vi "rmx13_tx - Copy (2).vi"() -> ()   [LabVIEW 2012]
uses:
  <vilib>/robotics/Steering/Steering Frame/NI_Robotics_Steering Frame.lvclass
  <vilib>/robotics/Steering/Wheel/NI_Robotics_Wheel.lvclass
  <vilib>/robotics/Utilities/Visualization/Steering Visualization/Steering Picture/NI_Robotics_Steering Picture.lvlib
  <vilib>/robotics/Steering/Fixed Wheel/Create Fixed Wheel.vi
  <vilib>/robotics/Steering/Fixed Wheel/NI_Robotics_Fixed Wheel.lvclass
  <vilib>/robotics/Steering/Differential Steering Frame/Create Differential Steering Frame.vi
  <vilib>/robotics/Steering/Differential Steering Frame/NI_Robotics_Differential Steering Frame.lvclass
  <vilib>/Utility/inputDevices.llb/closeKeyboard.vi
  <vilib>/robotics/Steering/Steering Frame/Apply Steering Frame Velocity to Wheels.vi
  <vilib>/Utility/inputDevices.llb/keyboardAcquire.vi
  <vilib>/robotics/Steering/Wheel/Wheel Parameters.ctl
  <vilib>/robotics/Steering/Wheel/Rotation Direction.ctl
panel:
  in  "Tab Control":enum32{"Front Panel", "Error Control"}(tab)
  in  "Boolean 2":bool
  in  "Boolean":bool
  out "Total Elapsed Time  (HH:MM:SS)":dbl format="%<%H:%M:%S%2u>t"
  out "hup":bool
  out "hdown":bool
  out "xfwd":bool
  out "xback":bool
  out "xdown":bool
  out "xup":bool
  out "right":bool
  out "left":bool
  out "down":bool
  out "up":bool
  out "right motor":dbl(knob) scale=-255.0..255.0
  out "left motor":dbl(knob) scale=-255.0..255.0
  out "Right":dbl=7.0 format="%#.2g"
  out "Left":dbl=3.0 format="%#.2g"
  out "picture":picture
  out "x-dir":string="a"
  out "bot-dir":string="a"
  out "x-state":string="a"
  out "h-state":string="a"
  out "error out":errorcluster
  in  "Horizontal Axis AI Pin":u8
  out "Out":dbl
  out "tx_string":string
  out "bytes written":i32
  # "Left Motor"
  # "Right Motor"
  # "Excavator State"
  # "Excavator Direction"
  # "Elapsed Time"
  # "Start/Stop"
  # "Bot Direction"
  # "Hopper State"
  # "Dump Position"
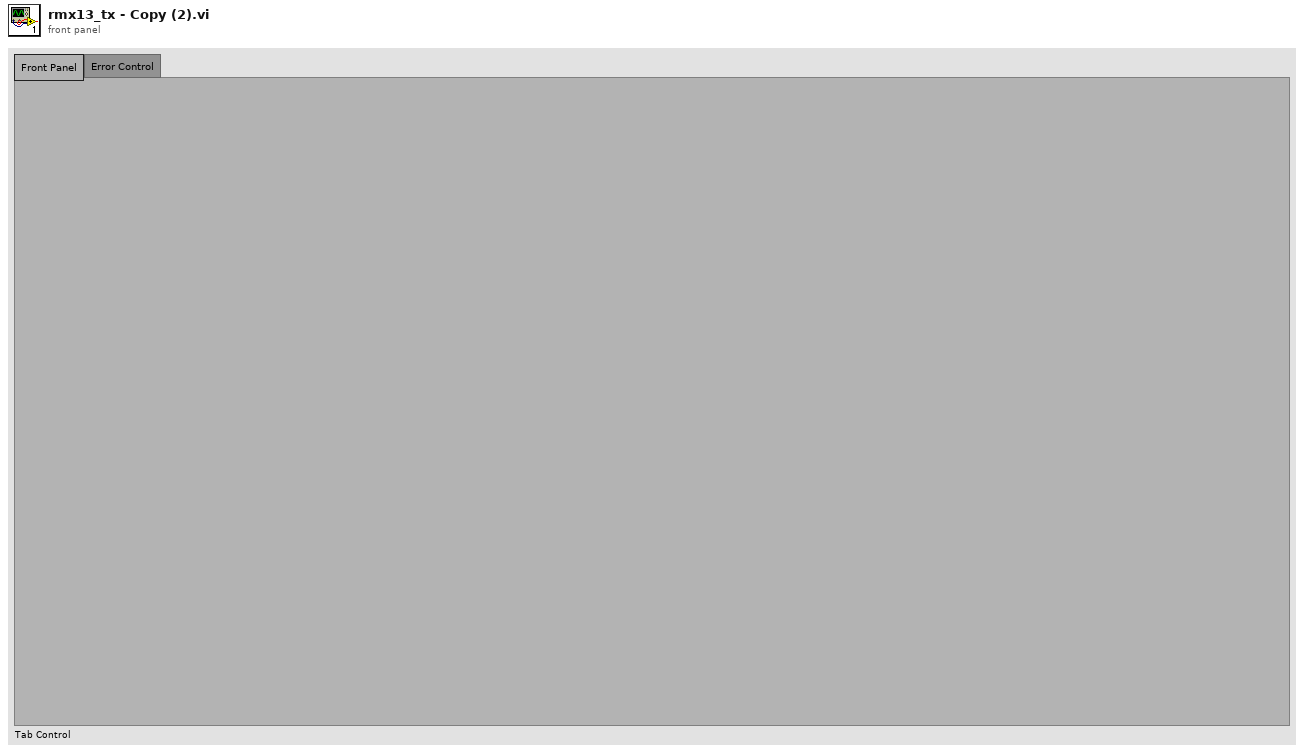
[diagram p1: front panel]
types:
  T1 = typedef "NI_Robotics_Wheel.lvclass/Wheel Parameters.ctl" = cluster{"wheel radius":dbl, "gear ratio":dbl, "forward rotation direction":T2}
  T2 = typedef "NI_Robotics_Wheel.lvclass/Rotation Direction.ctl" = u16
  T3 = cluster{"fixed wheel out":refnum<class "NI_Robotics_Fixed Wheel.lvclass">, "fixed wheel out":refnum<class "NI_Robotics_Fixed Wheel.lvclass">}
  T4 = typedef "LVBoundsTypeDef.ctl" = cluster{"Width":u32, "Height":u32}
  T5 = enum16{"0", "1", "2", "3", "4", "5", "6", "7", "8", "9", "A", "B", "C", "D", "E", "F", "G", "H", "I", "J", "K", "L", "M", "N", "O", "P", "Q", "R", "S", "T", "U", "V", "W", "X", "Y", "Z", "F1", "F2", "F3", "F4", "F5", "F6", "F7", "F8", "F9", "F10", "F11", "F12", "F13", "F14", "F15", "ADD", "BACK", "BACKSLASH", "CAPITAL", "COMMA", "DECIMAL", "DELETE", "DIVIDE", "DOWN", "END", "EQUALS", "ESCAPE", "GRAVE (`)", "HOME", "INSERT", "LBRACKET", "LCONTROL", "LEFT", "L ALT", "LSHIFT", "LWIN", "MINUS", "MULTIPLY", "NEXT", "NUMLOCK", "NUMPAD_0", "NUMPAD_1", "NUMPAD_2", "NUMPAD_3", "NUMPAD_4", "NUMPAD_5", "NUMPAD_6", "NUMPAD_7", "NUMPAD_8", "NUMPAD_9", "PAUSE", "PERIOD", "PRIOR (PG UP)", "RBRACKET", "RCONTROL", "RETURN", "RIGHT", "R ALT", "RSHIFT", "RWIN", "SCROLL", "SEMICOLON", "SLASH", "SPACE", "SUBTRACT", "TAB", "UP", "ENTER (num pad)", "' (quote)"}[]
  T6 = cluster{"up":bool, "down":bool, "left":bool, "right":bool, "xup":bool, "xdown":bool, "hup":bool, "hdown":bool, "xfwd":bool, "xback":bool}
  T7 = cluster{"bot_dir":string, "x-state":string, "h-state":string, "x-dir":string}
  T8 = typedef "NI_Robotics_Wheel.lvclass/Wheel State.ctl" = cluster{"wheel name":string, "forward angular velocity":dbl, "caster angular velocity":dbl, "caster wheel angle (rad)":dbl, "steering angle (rad)":dbl}
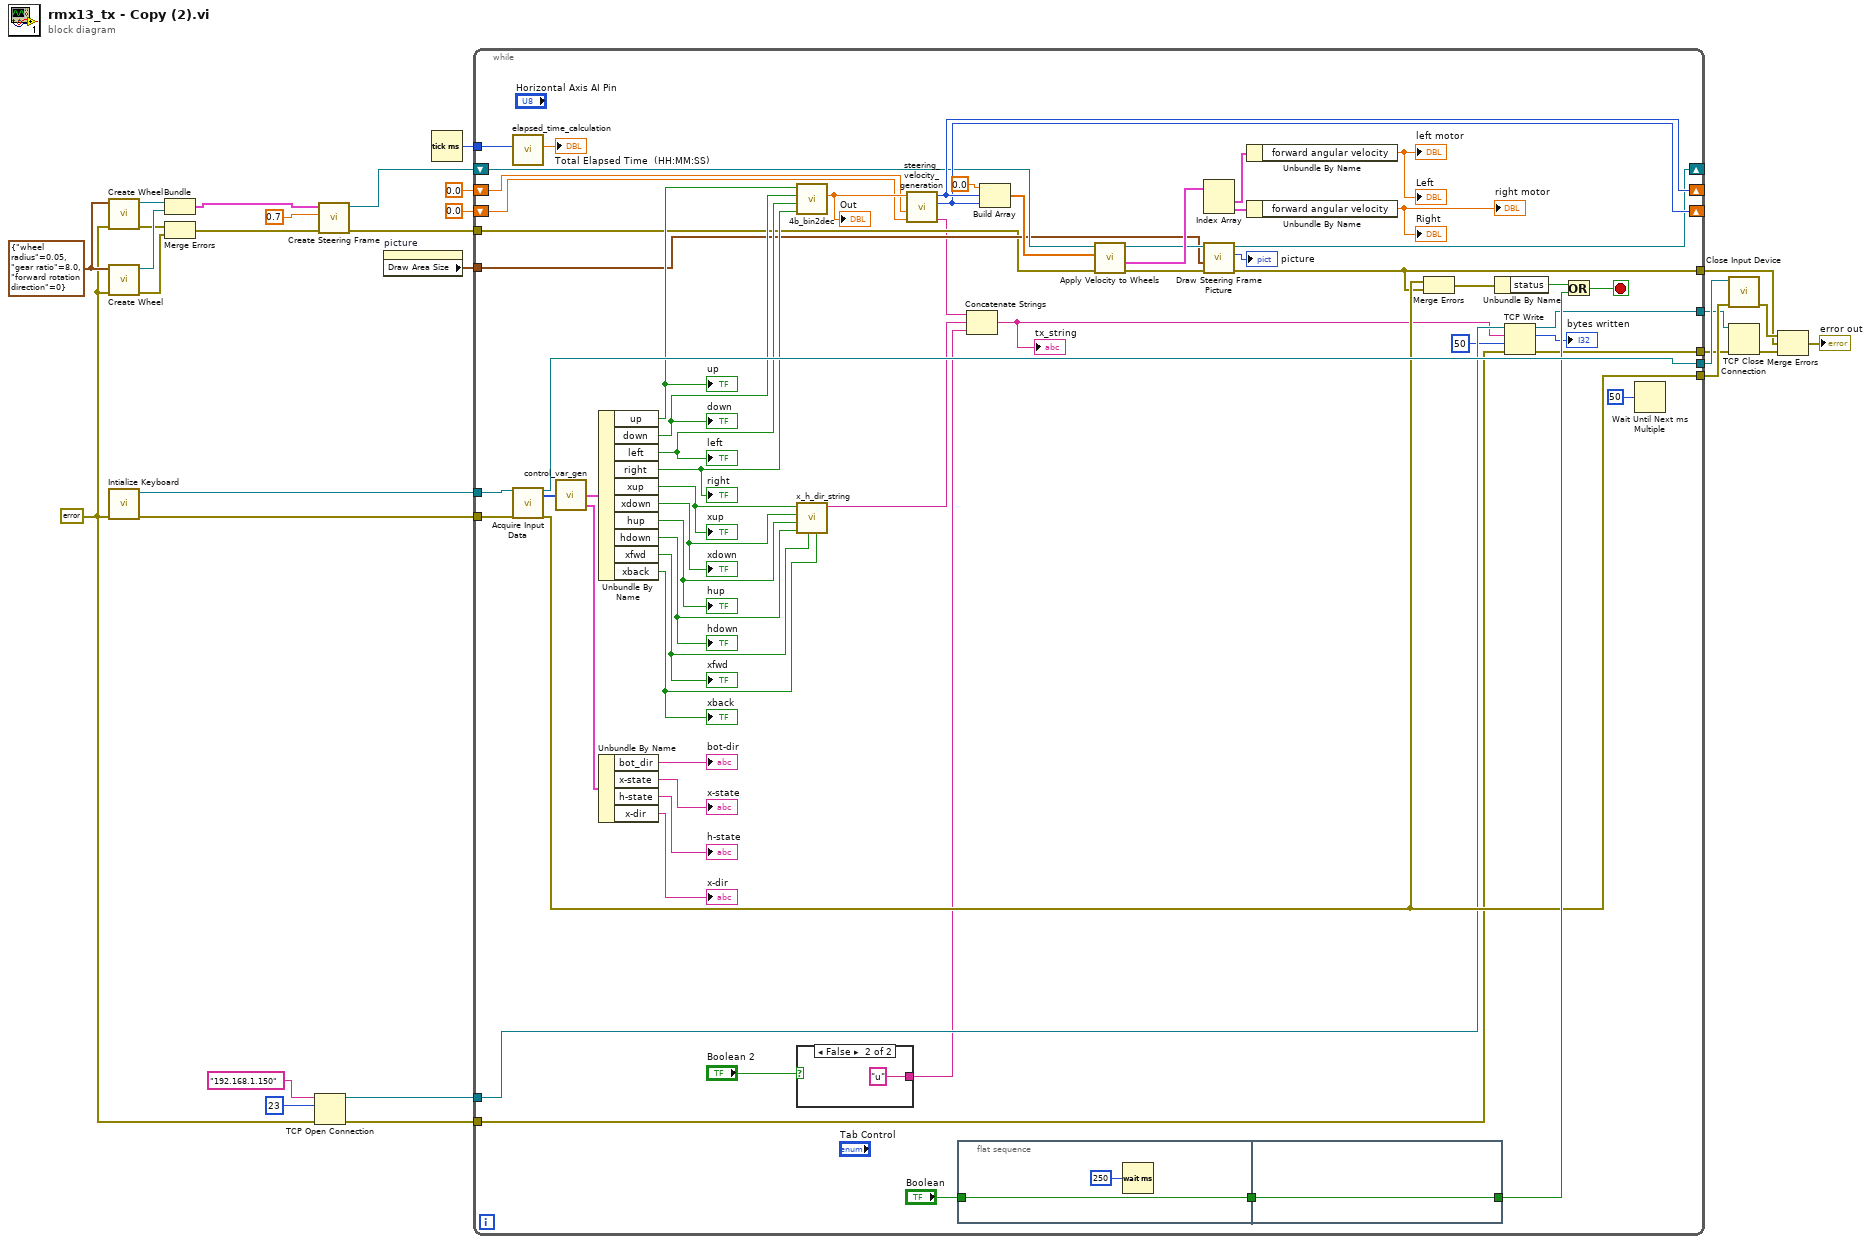
[diagram p0: block diagram]
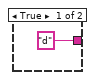
[diagram p2: hidden frame]
diagram:
  w1 = errorcluster {"status"=FALSE, "code"=0, "source"=""} ("error in")
  w19 = T1 {"wheel radius"=0.05, "gear ratio"=8.0, "forward rotation direction"=0} ("wheel parameters")
  n1 = call-poly <vilib>:"Create Wheel.vi"("error in (no error)"=w1, "wheel parameters"=w19) -> ("error out"=w18:errorcluster, "fixed wheel out"=w22:refnum<class "NI_Robotics_Fixed Wheel.lvclass">)  [unwired: 8 in]
  n2 = call-poly <vilib>:"Create Wheel.vi"("error in (no error)"=w1, "wheel parameters"=w19) -> ("error out"=w17:errorcluster, "fixed wheel out"=w21:refnum<class "NI_Robotics_Fixed Wheel.lvclass">)  [unwired: 8 in]
  n3 = call <vilib>:"Intialize Keyboard.vi"("error in (no error)"=w1) -> ("error out"=w28:errorcluster, "device ID"=w29:refnum<k1>)  [unwired: 9 in]
  n4 = Bundle("fixed wheel out"=w22, "fixed wheel out"=w21) -> (w20:T3)  [unwired: 1 in]
  n5 = Merge Errors(w18, w17) -> (w16:errorcluster)
  n6 = TCP Open Connection(address="192.168.1.150", remote port or service name=u16 23, error in (no error)=w1) -> (connection ID=w5:refnum<k5>, error out=w6:errorcluster)  [unwired: 2 in]
  n7 = call-poly <vilib>:"Create Steering Frame.vi"("error in (no error)"=w16, "wheel separation"=0.7, "wheels"=w20) -> ("error out"=w9:errorcluster, "differential steering frame out"=w11:refnum<class "NI_Robotics_Differential Steering Frame.lvclass">)  [unwired: 7 in]
  n8 = property on="picture" class="Pict"() -> ("Draw Area Size"=w10:T4)  [unwired: 2 in, 2 out]
  n9 = Tick Count (ms)() -> (millisecond timer value=w25:u32)
  n10 = while {
    tunnel: w29 -> [w90]
    tunnel: w28 -> [w89]
    tunnel: [w86] -> w27
    tunnel: [w67] -> w26
    tunnel: w25 -> [w59]
    shift-right: [w61] -> _
    shift-left: 0.0 -> [w63]
    shift-right: [w60] -> _
    shift-left: 0.0 -> [w62]
    tunnel: [w65] -> w13
    shift-right: [w52] -> _
    shift-left: w11 -> [w53]
    tunnel: w10 -> [w50]
    tunnel: w9 -> [w49]
    tunnel: w6 -> [w38]
    tunnel: w5 -> [w37]
    tunnel: [w33] -> w4
    tunnel: [w32] -> w3
    stop <- w68 stop-if-true
    n11 = call "elapsed_time_calculation.vi"("initial time"=w59) -> ("elapsed time"=→"Total Elapsed Time  (HH:MM:SS)":dbl)  [unwired: 10 in]
    n12 = call-poly <vilib>:"Acquire Input Data.vi"("device ID"=w90, "error in (no error)"=w89) -> ("device ID"=w86:refnum<k1>, "keys pressed"=w85:T5, "error out"=w67:errorcluster)  [unwired: 15 in]
    n13 = call "control_var_gen.vi"("keys pressed"=w85) -> ("out_panel"=w84:T6, "out_error"=w83:T7)  [unwired: 5 in]
    n14 = Unbundle By Name(w84) -> ("up"=w57:bool, "down"=w56:bool, "left"=w55:bool, "right"=w54:bool, "xup"=w46:bool, "xdown"=w45:bool, "hup"=w44:bool, "hdown"=w43:bool, "xfwd"=w42:bool, "xback"=w41:bool)
    "up" <- w57
    "down" <- w56
    "left" <- w55
    "right" <- w54
    "xup" <- w46
    "xdown" <- w45
    "hup" <- w44
    "hdown" <- w43
    "xfwd" <- w42
    "xback" <- w41
    n15 = Unbundle By Name(w83) -> ("bot_dir"=→"bot-dir":string, "x-state"=→"x-state":string, "h-state"=→"h-state":string, "x-dir"=→"x-dir":string)
    n16 = call "4b_bin2dec.vi"("Right"=w54, "Left"=w55, "Down"=w56, "Up"=w57) -> ("Out"=w64:dbl)  [unwired: 7 in]
    "Out" <- w64
    n17 = call "x_h_dir_string.vi"("xback"=w41, "xfwd"=w42, "hdown"=w43, "hup"=w44, "xdown"=w45, "xup"=w46) -> ("x_h_dir"=w39:string)  [unwired: 5 in]
    n18 = case shown="False" "Boolean 2" {
      tunnel: ["d" "u"] -> w30
      frame True {
      }
      frame False {
      }
    }
    n19 = call "steering_velocity_generation.vi"("angular velocity"=w62, "forward velocity"=w63, "bool-to-dec value"=w64) -> ("motor_control_sig"=w40:string, "angular velocity 2"=w60:i32, "forward velocity 2"=w61:i32)  [unwired: 6 in]
    n20 = flat-sequence {
      tunnel: "Boolean" -> [w93]
      tunnel: [w93] -> w88
      tunnel: [w95] -> w69
      tunnel: w88 -> [w95]
      frame #0 {
        n21 = Wait (ms)(milliseconds to wait=u32 250) -> ()  [unwired: 1 out]
      }
      frame #1 {
      }
    }
    n22 = Concatenate Strings(w40, w39, w30) -> (w35:string)
    "tx_string" <- w35
    n23 = Build Array(0.0 ("element"), w61, w60) -> (w73:dbl[])
    n24 = call-poly <vilib>:"Apply Velocity to Wheels.vi"("error in (no error)"=w49, "steering frame velocity"=w73, "steering frame in"=w53) -> ("error out"=w70:errorcluster, "calculated wheel states"=w72:T8[], "steering frame out"=w71:refnum<class "NI_Robotics_Differential Steering Frame.lvclass">)  [unwired: 5 in, 1 out]
    n25 = Index Array(array=w72) -> (element #1=w74:T8, element #2=w75:T8)  [unwired: 2 in]
    n26 = call <vilib>:"Draw Steering Frame Picture.vi"("error in (no error)"=w70, "picture draw area size (pixels)"=w50, "steering frame in"=w71) -> ("error out"=w65:errorcluster, "picture out"=→"picture":picture, "steering frame out"=w52:refnum<class "NI_Robotics_Differential Steering Frame.lvclass">)  [unwired: 6 in]
    n27 = Unbundle By Name(w74) -> ("forward angular velocity"=→"Left" →"left motor":dbl)
    n28 = Unbundle By Name(w75) -> ("forward angular velocity"=→"Right" →"right motor":dbl)
    n29 = Merge Errors(w67, w65) -> (w66:errorcluster)
    n30 = Unbundle By Name(w66) -> ("status"=w76:bool)
    n31 = TCP Write(connection ID=w37, data in=w35, error in (no error)=w38, 9:50 ("timeout ms (25000)")) -> (connection ID out=w33:refnum<k5>, bytes written=→"bytes written":i32, error out=w32:errorcluster)
    n32 = Or(x=w76, y=w69) -> (x .or. y?=w68:bool)
    n33 = Wait Until Next ms Multiple(millisecond multiple=u32 50) -> ()  [unwired: 1 out]
  }
  n34 = call-poly <vilib>:"Close Input Device.vi"("error in (no error)"=w26, "device ID"=w27) -> ("error out"=w24:errorcluster)  [unwired: 8 in]
  n35 = TCP Close Connection(connection ID=w4, error in (no error)=w3) -> (error out=w2:errorcluster)  [unwired: 1 in, 1 out]
  n36 = Merge Errors(w24, w13, w2) -> (→"error out":errorcluster)
